vi "Construct_2DGaussian_Fitting.vi"(8 "Error In":errorcluster, 11 "OD(2D)":dbl[][](array[numeric])) -> (0 "error out":errorcluster, 1 "best fit parameters":dbl[](array[numeric]), 2 "Elapsed time in ms":u32, 3 "Fit Image":dbl[][](graph))   [LabVIEW 2016]
uses:
  <vilib>/gmath/NumericalOptimization/Nonlinear Curve Fit LM.vi
  <vilib>/gmath/NI_Gmath.lvlib
panel:
  out "Initial guesses":dbl[](array[numeric])
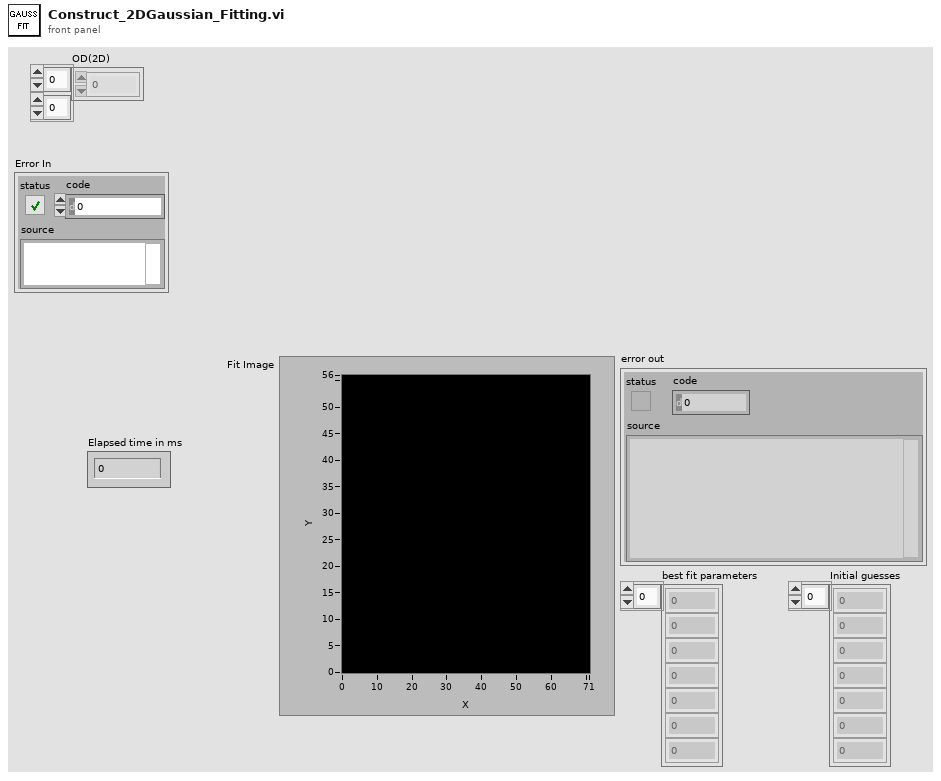
[diagram p1: front panel]
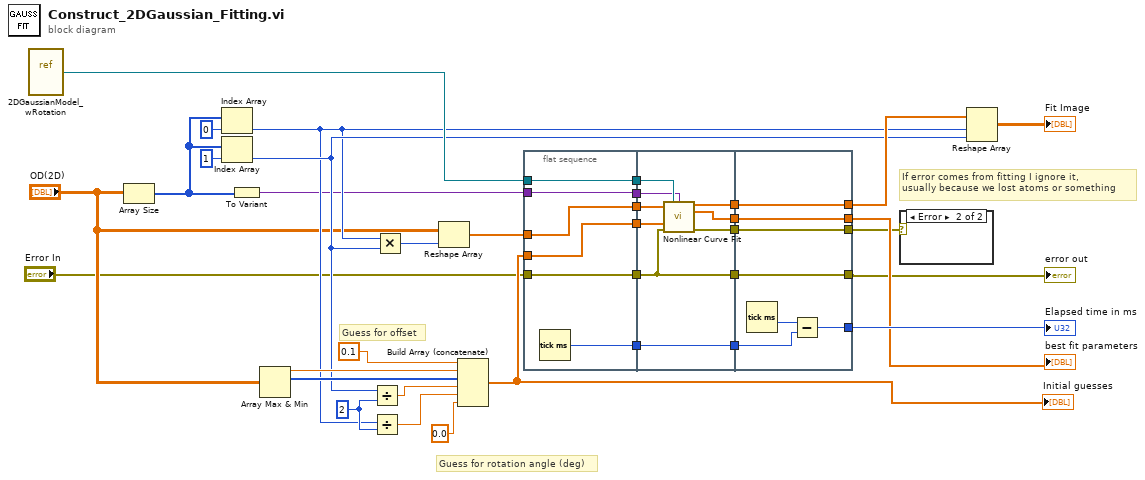
[diagram p0: block diagram]
diagram:
  w30 = 2
  # "Guess for rotation angle (deg)"
  # "Guess for offset"
  # "If error comes from fitting I ignore it, \nusually because we lost atoms or something"
  n1 = vi-ref "2DGaussianModel_wRotation.vi"() -> (w35:refnum<vi>)
  n2 = Array Size(array="OD(2D)") -> (size(s)=w11:i32[])
  n3 = Index Array(array=w11, index=0) -> (element=w14:i32)
  n4 = Index Array(array=w11, index=1) -> (element=w15:i32)
  n5 = To Variant(anything=w11) -> (Variant=w9:variant)
  n6 = Array Max & Min(array="OD(2D)") -> (max value=w31:dbl, max index (indices)=w32:i32[])  [unwired: 2 out]
  n7 = Divide(x=w15, y=w30) -> (x/y=w29:dbl)
  n8 = Divide(x=w14, y=w30) -> (x/y=w28:dbl)
  n9 = Multiply(x=w14, y=w15) -> (x*y=w36:i32)
  n10 = Reshape Array("OD(2D)", w36) -> (w12:dbl[])
  n11 = Build Array (concatenate)(0.1, w31, w32, w29, w28, 0.0 ("element")) -> (w18:dbl[])
  "Initial guesses" <- w18
  n12 = flat-sequence {
    tunnel: w35 -> [w42]
    tunnel: [w42] -> w27
    tunnel: w12 -> [w39]
    tunnel: [w41] -> w26
    tunnel: w18 -> [w41]
    tunnel: [w40] -> w25
    tunnel: [w39] -> w24
    tunnel: [w38] -> w10
    tunnel: w9 -> [w38]
    tunnel: [w37] -> w7
    tunnel: "Error In" -> [w37]
    tunnel: w27 -> [w51]
    tunnel: w26 -> [w50]
    tunnel: [w49] -> w23
    tunnel: [w48] -> w22
    tunnel: w25 -> [w47]
    tunnel: [w47] -> w21
    tunnel: w24 -> [w45]
    tunnel: [w46] -> w20
    tunnel: w10 -> [w44]
    tunnel: w7 -> [w43]
    tunnel: [w43] -> w4
    tunnel: [w57] -> w33
    tunnel: [w58] -> w8
    tunnel: w23 -> [w58]
    tunnel: w22 -> [w57]
    tunnel: w21 -> [w55]
    tunnel: [w54] -> w5
    tunnel: w20 -> [w54]
    tunnel: [w53] -> w19
    tunnel: [w52] -> w3
    tunnel: w4 -> [w52]
    frame #0 {
      n13 = Tick Count (ms)() -> (millisecond timer value=w40:u32)
    }
    frame #1 {
      n14 = call-poly <vilib>:"Nonlinear Curve Fit.vi"("Y"=w45, "f(x,a)"=w51, "data"=w44, "initial parameters"=w50, "error in (no error)"=w43) -> ("best nonlinear fit"=w48:dbl[], "best fit parameters"=w49:dbl[], "error out"=w46:errorcluster)  [unwired: 5 in, 3 out]
    }
    frame #2 {
      n15 = Tick Count (ms)() -> (millisecond timer value=w56:u32)
      n16 = Subtract(x=w56, y=w55) -> (x-y=w53:u32)
    }
  }
  n17 = case shown="Error" w5 {
    frame No Error {
    }
    frame Error {
    }
  }
  n18 = Reshape Array(w33, w14, w15) -> (→"Fit Image":dbl[][])
  "error out" <- w3
  "Elapsed time in ms" <- w19
  "best fit parameters" <- w8
